vi "123.vi"(11 "HealthAndStatusDataFIFO in":refnum<class "HealthAndStatusDataFIFO.lvclass">) -> (2 "FPGAReference":refnum<k20>, 3 "HealthAndStatusDataFIFO out":refnum<class "HealthAndStatusDataFIFO.lvclass">)   [LabVIEW 2016]
uses:
  HealthAndStatusDataFIFO.lvclass
  D:/Code/ts_M1M3Support/Common_RT_FPGA/IReadU32FIFO/IReadU32FIFO.lvclass
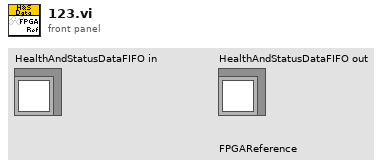
[diagram p1: front panel]
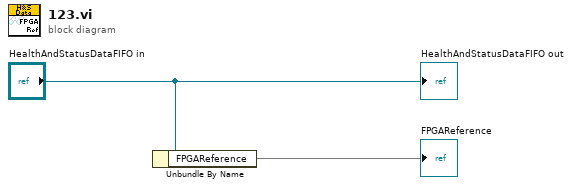
[diagram p0: block diagram]
diagram:
  n1 = Unbundle By Name("HealthAndStatusDataFIFO in") -> ("FPGAReference"=→"FPGAReference")
  "HealthAndStatusDataFIFO out" <- "HealthAndStatusDataFIFO in"
